vi "XML readSamplesFromXML.getAttributes.vi"(10 "Sample XML":string, 11 "Sample in":T1) -> (3 "Sample out":T1)   [LabVIEW 2011]
uses:
  Controls/PIM.API.Response.Samples.ctl
  iQA Sweep Behavior.ctl
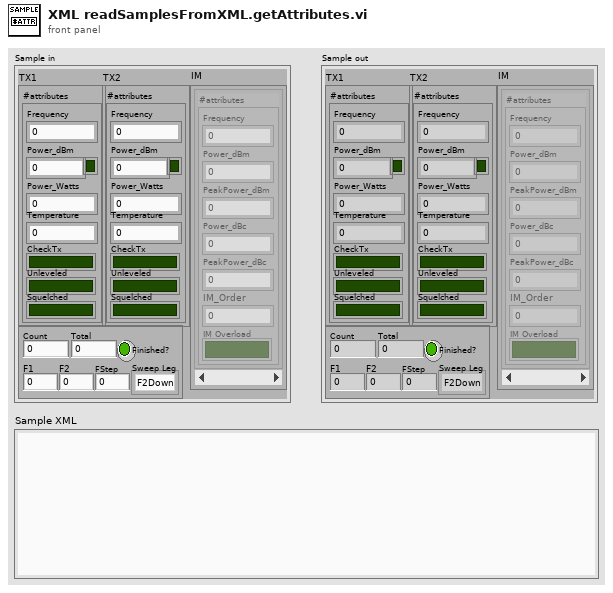
[diagram p1: front panel]
types:
  T1 = typedef "PIM.API.Response.Samples.ctl" = cluster{"TX1":cluster{"#attributes":cluster{"Frequency":dbl, "Power_dBm":dbl, "Power_Watts":dbl, "CheckTx":bool, "Unleveled":bool, "Squelched":bool, "Temperature":dbl, "ToneOn":bool}}, "TX2":cluster{"#attributes":cluster{"Frequency":dbl, "Power_dBm":dbl, "Power_Watts":dbl, "CheckTx":bool, "Unleveled":bool, "Squelched":bool, "Temperature":dbl, "ToneOn":bool}}, "IM":cluster{"#attributes":cluster{"Frequency":dbl, "Power_dBm":dbl, "PeakPower_dBm":dbl, "Power_dBc":dbl, "PeakPower_dBc":dbl, "IM_Order":u8, "IM Overload":bool}}[], "#attributes":cluster{"Count":u32, "Total":u32, "Finished?":bool, "Sweep Leg":T2, "F1":dbl, "F2":dbl, "FStep":dbl}}
  T2 = typedef "iQA Sweep Behavior.ctl" = enum16{"F2Down", "F1Up", "RxMultiIM"}
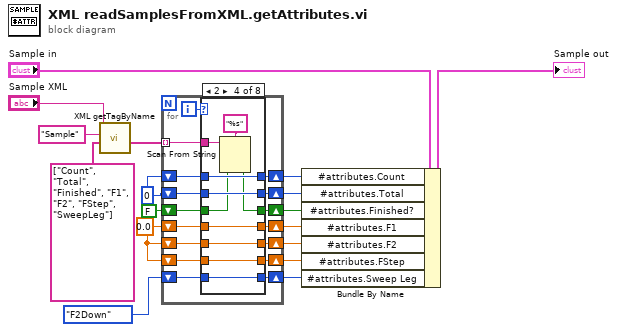
[diagram p0: block diagram]
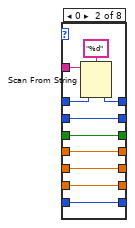
[diagram p3: hidden frame]
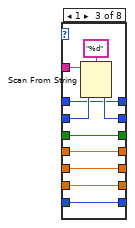
[diagram p4: hidden frame]
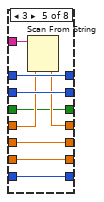
[diagram p5: hidden frame]
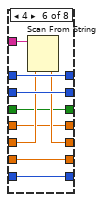
[diagram p6: hidden frame]
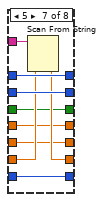
[diagram p7: hidden frame]
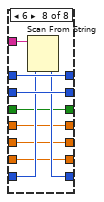
[diagram p8: hidden frame]
diagram:
  w6 = 0.0 ("#attributes.Total")
  w13 = u32 0 ("#attributes.Total")
  n1 = call "XML getTagByName.vi"("Get Attributes"=string[] ["Count", "Total", "Finished", "F1", "F2", "FStep", "SweepLeg"], "Tag Name"="Sample", "XML String"="Sample XML") -> ("Attribute Values"=w16:string[])  [unwired: 4 in, 4 out]
  n2 = for {
    shift-right: [w32] -> w15
    shift-left: w13 -> [w29]
    shift-right: [w31] -> w14
    shift-left: w13 -> [w30]
    shift-right: [w27] -> w12
    shift-left: FALSE -> [w28]
    tunnel: w16 -> [w26] mode=indexing
    shift-right: [w18] -> w5
    shift-left: w6 -> [w25]
    shift-right: [w19] -> w4
    shift-left: w6 -> [w24]
    shift-right: [w20] -> w3
    shift-left: w6 -> [w23]
    shift-right: [w21] -> w1
    shift-left: enum16{"F2Down", "F1Up"}."F2Down" ("#attributes.Sweep Leg") -> [w22]
    i -> [w33]
    n3 = case shown="2" w33 {
      tunnel: [w40 w49 w56 w68 w78 w87 w96 w105] -> w32
      tunnel: [w39 w47 w59 w69 w79 w88 w97 w106] -> w31
      tunnel: w30 -> [w39 w47 w58 w69 w79 w88 w97 w106]
      tunnel: w29 -> [w40 w48 w56 w68 w78 w87 w96 w105]
      tunnel: w28 -> [w38 w46 w57 w67 w71 w80 w89 w98]
      tunnel: [w38 w46 w57 w66 w71 w80 w89 w98] -> w27
      tunnel: w26 -> [_ w45 w55 w65 w77 w86 w95 w104]
      tunnel: w25 -> [w34 w41 w51 w61 w76 w81 w90 w99]
      tunnel: w24 -> [w35 w42 w52 w62 w72 w85 w91 w100]
      tunnel: w23 -> [w36 w43 w53 w63 w73 w82 w94 w101]
      tunnel: w22 -> [w37 w44 w54 w64 w74 w83 w92 w103]
      tunnel: [w37 w44 w54 w64 w74 w83 w92 w102] -> w21
      tunnel: [w36 w43 w53 w63 w73 w82 w93 w101] -> w20
      tunnel: [w35 w42 w52 w62 w72 w84 w91 w100] -> w19
      tunnel: [w34 w41 w51 w61 w75 w81 w90 w99] -> w18
      frame Default {
      }
      frame 0 {
        n4 = Scan From String(format string="%d", input string=w45, default 1=w48) -> (output 1=w49:u32)  [unwired: 2 in, 3 out]
      }
      frame 1 {
        n5 = Scan From String(format string="%d", input string=w55, default 1=w58) -> (output 1=w59:u32)  [unwired: 2 in, 3 out]
      }
      frame 2 {
        n6 = Scan From String(format string="%s", input string=w65, default 1=w67) -> (output 1=w66:bool)  [unwired: 2 in, 3 out]
      }
      frame 3 {
        n7 = Scan From String(input string=w77, default 1=w76) -> (output 1=w75:dbl)  [unwired: 3 in, 3 out]
      }
      frame 4 {
        n8 = Scan From String(input string=w86, default 1=w85) -> (output 1=w84:dbl)  [unwired: 3 in, 3 out]
      }
      frame 5 {
        n9 = Scan From String(input string=w95, default 1=w94) -> (output 1=w93:dbl)  [unwired: 3 in, 3 out]
      }
      frame 6 {
        n10 = Scan From String(input string=w104, default 1=w103) -> (output 1=w102:enum16{"F2Down", "F1Up"})  [unwired: 3 in, 3 out]
      }
    }
  }
  n11 = Bundle By Name(cluster="Sample in", "#attributes.Count"=w15, "#attributes.Total"=w14, "#attributes.Finished?"=w12, "#attributes.F1"=w5, "#attributes.F2"=w4, "#attributes.FStep"=w3, "#attributes.Sweep Leg"=w1) -> (→"Sample out":T1)
